vi "plot Unix to LV epoch.vi"(11 "Plot (unix)":T1) -> (3 "Plot (LV epoch)":cluster{dbl[], "Data":dbl[]})   [LabVIEW 2021, in "RocketPlot.lvlib"]
uses:
  RocketPlot.lvlib
  TypeDefs/plot datapoint.ctl
  3a8248cf-bec7-4c8d-a232-b35239452a92.vi
  6d88088e-0f8c-482f-b724-f15eac533201.vi
  <userlib>/bjustice/Ring Buffer for Time Series Data Strict Accessor/Unix time epoch/Unix_Epoch_in_Labview.vi
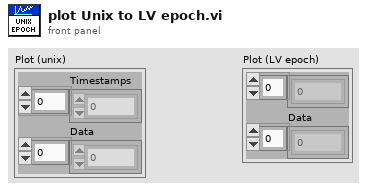
[diagram p1: front panel]
types:
  T1 = typedef "RocketPlot.lvlib/plot datapoint.ctl" = cluster{"Timestamps":u64[], "Data":dbl[]}
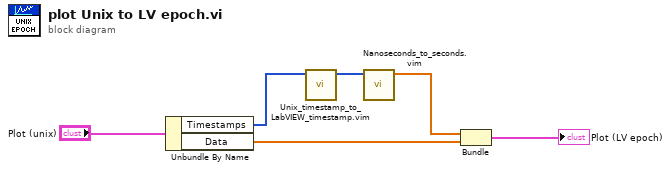
[diagram p0: block diagram]
diagram:
  n1 = Unbundle By Name("Plot (unix)") -> ("Timestamps"=w3:u64[], "Data"=w4:dbl[])
  n2 = call "Unix_timestamp_to_LabVIEW_timestamp.vim"("Unix timestamp (nanoseconds)"=w3) -> ("LabVIEW timestamp (nanoseconds)"=w2:u64[])  [unwired: 10 in]
  n3 = call "Nanoseconds_to_seconds.vim"("nanoseconds"=w2) -> ("seconds"=w1:dbl[])  [unwired: 10 in]
  n4 = Bundle("seconds"=w1, "Data"=w4) -> (→"Plot (LV epoch)":cluster{"seconds":dbl[], "Data":dbl[]})  [unwired: 1 in]
